vi "detrend_and_limit_cdb.vi"(8 "Parameters":T1, 11 "Input":cdb[](array[numeric])) -> (3 "Output":cdb[](array[numeric]))   [LabVIEW 2014]
uses:
  averaging_filter_params.ctl
  detrend_mode.ctl
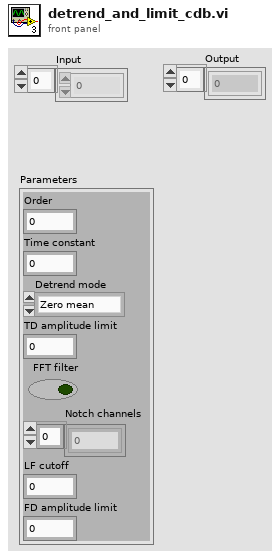
[diagram p1: front panel]
types:
  T1 = typedef "averaging_filter_params.ctl" = cluster{"Order":i32, "Time constant":dbl, "Detrend mode":T2, "TD amplitude limit":dbl, "FFT filter":bool, "Notch channels":i32[], "LF cutoff":i32, "FD amplitude limit":dbl}
  T2 = typedef "detrend_mode.ctl" = enum16{"Zero mean", "Linear", "Robust linear"}
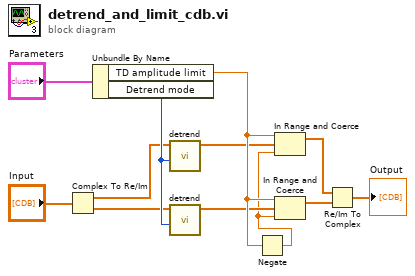
[diagram p0: block diagram]
diagram:
  n1 = Complex To Re/Im(x + iy="Input") -> (x=w5:dbl[], y=w7:dbl[])
  n2 = Unbundle By Name("Parameters") -> ("TD amplitude limit"=w11:dbl, "Detrend mode"=w12:T2)
  n3 = call "detrend.vi"("Detrend mode"=w12, "Input"=w5) -> ("Output"=w6:dbl[])  [unwired: 7 in, 2 out]
  n4 = call "detrend.vi"("Detrend mode"=w12, "Input"=w7) -> ("Output"=w8:dbl[])  [unwired: 7 in, 2 out]
  n5 = Negate(x=w11) -> (-x=w3:dbl)
  n6 = In Range and Coerce(upper limit=w11, x=w6, lower limit=w3) -> (coerced(x)=w1:dbl[])  [unwired: 1 out]
  n7 = In Range and Coerce(upper limit=w11, x=w8, lower limit=w3) -> (coerced(x)=w4:dbl[])  [unwired: 1 out]
  n8 = Re/Im To Complex(1:w4, 2:w1) -> (0:→"Output":cdb[])
